vi "Generator_a.vi"(0 "Stop":bool caption="Start/Stop") -> (4 "Generated_Data":dbl caption="Generated Data")   [LabVIEW 2023]
doc: "This VI continuously generate Data and push it to the Acquisition VI.\nTransfer of thet data happens under Global variable."
uses:
  <vilib>/numeric/Random Number (Range) DBL.vi
  Global_Variables/Generate_Data_Global.vi
panel:
  in  "Error_In":errorcluster
  out "Error_Out":errorcluster
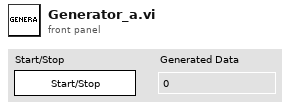
[diagram p1: front panel]
types:
  T1 = enum16{"Left Button", "Center Button", "Right Button", "Window Close"}
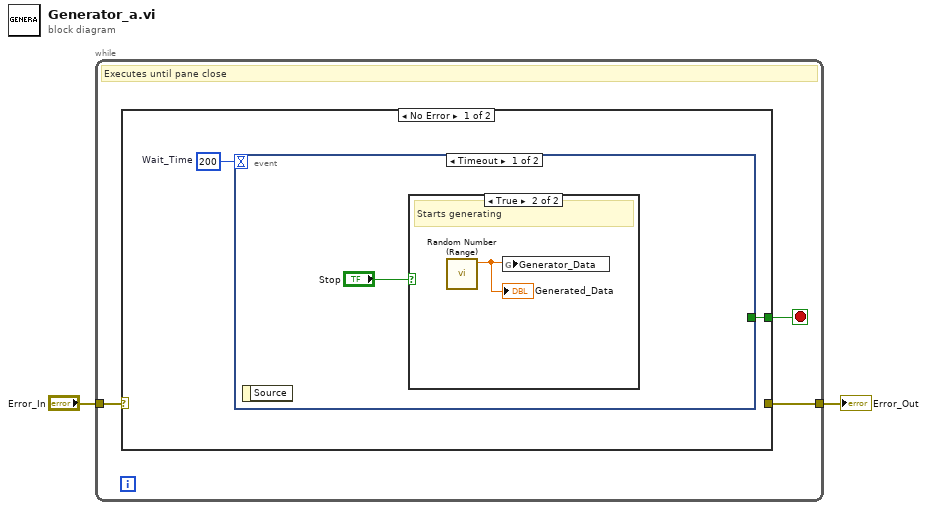
[diagram p0: block diagram]
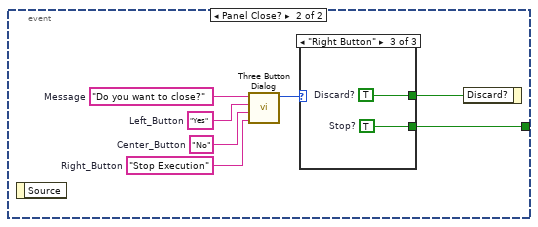
[diagram p3: hidden frame]
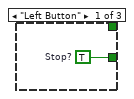
[diagram p4: hidden frame]
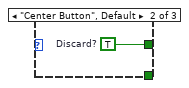
[diagram p5: hidden frame]
diagram:
  n1 = while {
    tunnel: [w4] -> w2
    tunnel: "Error_In" -> [w3]
    stop <- w5 stop-if-true
    # "Executes until pane close"
    n2 = case shown="No Error" w3 {
      selector: w3 -> [_ w21]
      tunnel: [w6 _] -> w5
      tunnel: [_ w21] -> w4
      frame No Error {
        w7 = 200  # Wait_Time
        n3 = event shown="[0] Timeout" {
          selector: _ -> [_ _]
          dyn-events: _ -> [_ _]
          timeout: w7 -> [_ _]
          tunnel: [_ w10] -> w6
          event Timeout {
            n4 = event-data() -> ()  [unwired: 1 in, 1 out]
            n5 = case shown="True" "Stop" {
              frame False {
                # "Stop generating"
              }
              frame True {
                # "Starts generating"
                n6 = call-poly <vilib>:"Random Number (Range).vi"() -> ("number"=w9:dbl)  [unwired: 11 in]
                "Generated_Data" <- w9
                n7 = global write "Generate_Data_Global.vi" "Generator_Data"(w9) -> ()
              }
            }
          }
          event Panel Close? {
            w13 = "Stop Execution"  # Right_Button
            w14 = "No"  # Center_Button
            w15 = "Yes"  # Left_Button
            w16 = "Do you want to close?"  # Message
            n8 = event-data() -> ()  [unwired: 1 in, 1 out]
            n9 = call <vilib>:"Three Button Dialog.vi"("Right Button Text (\"Cancel\")"=w13, "Center Button Text (\"No\")"=w14, "Left Button Text (\"Yes\")"=w15, "message"=w16) -> ("Which Button?"=w12:T1)  [unwired: 7 in]
            n10 = case shown="\"Right Button\"" w12 {
              tunnel: [_ w18 w19] -> w11
              tunnel: [w17 _ w20] -> w10
              frame "Left Button" {
                w17 = TRUE  # Stop?
              }
              frame "Center Button", Default {
                w18 = TRUE  # Discard?
              }
              frame "Right Button" {
                w19 = TRUE  # Discard?
                w20 = TRUE  # Stop?
              }
            }
            n11 = event-data("Discard?"=w11) -> ()  [unwired: 1 in, 1 out]
          }
        }
      }
      frame Error {
      }
    }
  }
  "Error_Out" <- w2
